vi "HW IO Get Connection.vi"(8 "error in (no error)":errorcluster, 9 "Port":u16=8833, 10 "Server":string="localhost") -> (0 "error out":errorcluster, 1 "API Port out":u16, 2 "API Server out":string, 3 "connection ID":refnum<k5>)   [LabVIEW 2011]
uses:
  HWIO Global.vi
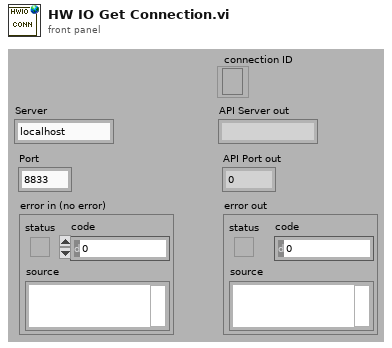
[diagram p1: front panel]
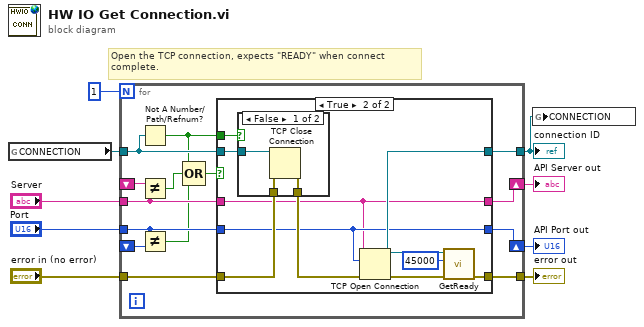
[diagram p0: block diagram]
diagram:
  # "Open the TCP connection, expects \"READY\" when connect\ncomplete."
  n1 = global read "HWIO Global.vi" "CONNECTION"() -> (w2:refnum<k5>)
  n2 = for {
    N: 1 -> [_]
    tunnel: "Server" -> [w16]
    tunnel: "Port" -> [w14]
    tunnel: "error in (no error)" -> [w21]
    tunnel: [w22] -> w5
    shift-right: [w19] -> w4
    shift-left: _ -> [w17]
    shift-right: [w20] -> w3
    shift-left: _ -> [w15]
    tunnel: w2 -> [w18]
    tunnel: [w23] -> w1
    n3 = Not A Number/Path/Refnum?(number/path/refnum=w18) -> (NaN/Path/Refnum?=w10:bool)
    n4 = Not Equal?(x=w17, y=w16) -> (x != y?=w13:bool)
    n5 = Not Equal?(x=w14, y=w15) -> (x != y?=w12:bool)
    n6 = Compound Arithmetic op=OR(w10, w13, w12) -> (w11:bool)
    n7 = case shown="True" w11 {
      tunnel: w18 -> [w26 w34]
      tunnel: w16 -> [w25 w29]
      tunnel: w14 -> [w24 w30]
      tunnel: [w26 w35] -> w23
      tunnel: [w27 w32] -> w22
      tunnel: w21 -> [w27 w31]
      tunnel: [w24 w30] -> w20
      tunnel: [w25 w29] -> w19
      tunnel: w10 -> [_ w28]
      frame False {
      }
      frame True {
        n8 = case shown="False" w28 {
          tunnel: w34 -> [w40 _]
          tunnel: [w39 w41] -> w33
          tunnel: w31 -> [w38 w41]
          frame False {
            n9 = TCP Close Connection(connection ID=w40, error in (no error)=w38) -> (error out=w39:errorcluster)  [unwired: 1 in, 1 out]
          }
          frame True {
          }
        }
        n10 = TCP Open Connection(address=w29, remote port or service name=w30, error in (no error)=w33) -> (connection ID=w35:refnum<k5>, error out=w36:errorcluster)  [unwired: 2 in]
        n11 = call "GetReady.vi"("error in (no error)"=w36, "Timeout, (10000 ms)"=45000, "connection ID"=w35) -> ("error out"=w32:errorcluster)  [unwired: 4 out]
      }
    }
  }
  "connection ID" <- w1
  "error out" <- w5
  "API Server out" <- w4
  "API Port out" <- w3
  n12 = global write "HWIO Global.vi" "CONNECTION"(w1) -> ()
